vi "keycommand.vi"(0 "MoAgSy_GPG in":refnum<class "MoAgSy_GPG.lvclass">, 1 "options file":path, 3 "keyringfile":path, 4 "Sec keyringfile":path, 5 "targetfile":path, 7 "error in (no error)":errorcluster, 8 "key-id":string, 9 "SecKey (f)":bool, 10 "Trust DB":path, 12 "Enum":T1(ring), 14 "overwrite? (t)":bool=TRUE) -> (13 "return code":i32, 15 "standard error":string, 16 "data error?":bool, 17 "standard output":string, 18 "dup Trust DB":path, 20 "MoAgSy_GPG out":refnum<class "MoAgSy_GPG.lvclass">, 21 "dup options file":path, 23 "dup keyringfile":path, 24 "dup Sec keyringfile":path, 25 "dup targetfile":path, 27 "error out":errorcluster)   [LabVIEW 2009, in "MoAgSy.lvlib" / "MoAgSy_GPG.lvclass"]
doc: "Executes following commandline tools of the GnuPG:\ndelete key\nexport key\nimport key"
uses:
  MoAgSy_GPG.lvclass
  HGF_GPG/HGF_GPG.lvclass/HGF_GPG.lvclass
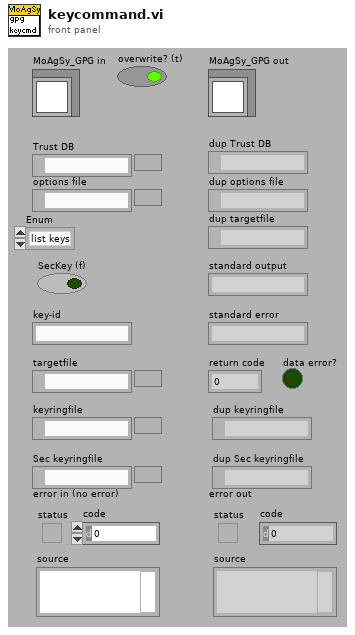
[diagram p1: front panel]
types:
  T1 = enum16{"list keys", "export", "import", "delete"}
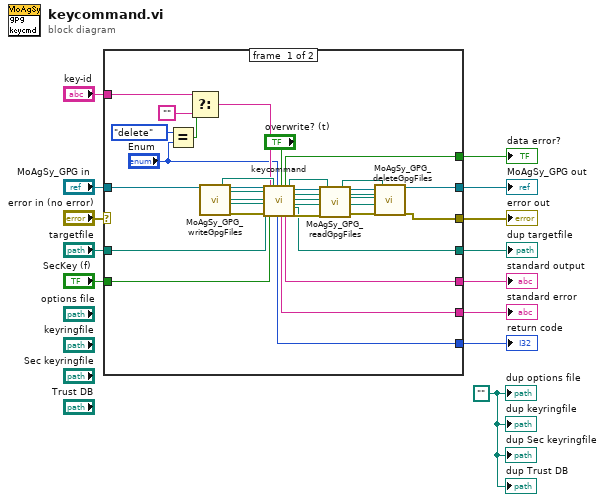
[diagram p0: block diagram]
diagram:
  w4 = path ""
  n1 = case shown="No Error" "error in (no error)" {
    selector: "error in (no error)" -> [_ w51]
    tunnel: "MoAgSy_GPG in" -> [w40 w49]
    tunnel: "SecKey (f)" -> [w47 _]
    tunnel: [w46 _] -> w11
    tunnel: [w45 _] -> w10
    tunnel: [w44 _] -> w9
    tunnel: [w43 _] -> w8
    tunnel: [w32 w49] -> w7
    tunnel: [w42 w50] -> w6
    tunnel: [w31 w51] -> w5
    tunnel: "targetfile" -> [w41 w50]
    tunnel: "key-id" -> [w19 _]
    frame #0 {
      n2 = Equal?(x=T1."delete" ("y"), y="Enum") -> (x = y?=w17:bool)
      n3 = Select(t=w19, s=w17, f="") -> (s? t:f=w16:string)
      n4 = call "MoAgSy_GPG_writeGpgFiles.vi"("MoAgSy_GPG"=w40) -> ("trust db file"=w36:path, "dup MoAgSy_GPG"=w39:refnum<class "MoAgSy_GPG.lvclass">, "options file"=w35:path, "keyring file"=w34:path, "sec keyring file"=w33:path, "error out"=w38:errorcluster)  [unwired: 1 in, 12 out]
      n5 = call-parent "keycommand.vi"("HGF_GPG in"=w39, "options file"=w35, "keyringfile"=w34, "Sec keyringfile"=w33, "targetfile"=w41, "error in (no error)"=w38, "key-id"=w16, "SecKey (f)"=w47, "Trust DB"=w36, "Enum"="Enum", "overwrite? (t)"="overwrite? (t)") -> ("return code"=w46:i32, "standard error"=w45:string, "data error?"=w44:bool, "standard output"=w43:string, "dup Trust DB"=w28:path, "HGF_GPG out"=w30:refnum<class "MoAgSy_GPG.lvclass">, "dup options file"=w26:path, "dup keyringfile"=w25:path, "dup Sec keyringfile"=w24:path, "dup targetfile"=w42:path, "error out"=w48:errorcluster)  [unwired: 6 out]
      n6 = call "MoAgSy_GPG_readGpgFiles.vi"("MoAgSy_GPG in"=w30, "options file"=w26, "keyring file"=w25, "sec keyring file"=w24, "error in (no error)"=w48, "trust db file"=w28) -> ("dup trust db file"=w27:path, "MoAgSy_GPG out"=w29:refnum<class "MoAgSy_GPG.lvclass">, "dup options file"=w23:path, "dup keyring file"=w22:path, "dup sec keyring file"=w21:path, "error out"=w20:errorcluster)  [unwired: 8 out]
      n7 = call "MoAgSy_GPG_deleteGpgFiles.vi"("MoAgSy_GPG"=w29, "options file"=w23, "keyringfile"=w22, "Sec keyringfile"=w21, "error in (no error)"=w20, "Trust DB"=w27) -> ("dup MoAgSy_GPG"=w32:refnum<class "MoAgSy_GPG.lvclass">, "error out"=w31:errorcluster)  [unwired: 12 out]
    }
    frame #1 {
    }
  }
  "error out" <- w5
  "MoAgSy_GPG out" <- w7
  "dup targetfile" <- w6
  "data error?" <- w9
  "standard output" <- w8
  "standard error" <- w10
  "return code" <- w11
  "dup keyringfile" <- w4
  "dup options file" <- w4
  "dup Sec keyringfile" <- w4
  "dup Trust DB" <- w4
